vi "bh3_create_package.vi"(10 "Payload":u8[](array[numeric]) format="%02x", 11 "msg_ID":u8 format="%02x") -> (2 "package byte array":u8[](array[numeric]) format="%02x", 3 "package string":string)   [LabVIEW 2013]
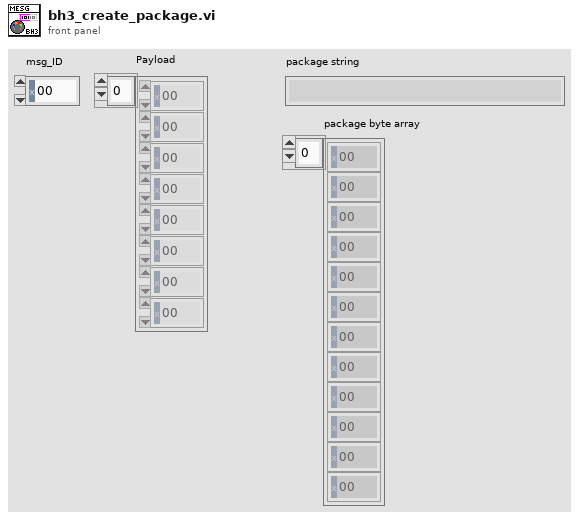
[diagram p1: front panel]
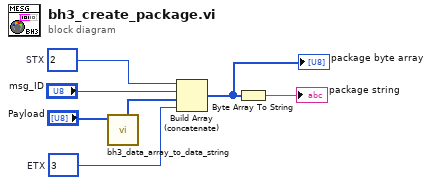
[diagram p0: block diagram]
diagram:
  w6 = u8 3  # ETX
  w7 = u8 2  # STX
  n1 = call "bh3_data_array_to_data_string.vi"("payload"="Payload") -> ("DLC_payload_CRC bytes"=w1:u8[])  [unwired: 6 in, 4 out]
  n2 = Build Array (concatenate)(w7, "msg_ID", w1, w6) -> (w4:u8[])
  "package byte array" <- w4
  n3 = Byte Array To String(unsigned byte array=w4) -> (string=→"package string":string)
